vi "multichat.vi"() -> ()   [LabVIEW 2016]
uses:
  <vilib>/httpClient/POSTBuffer.vi
  <vilib>/httpClient/LabVIEWHTTPClient.lvlib
panel:
  in  "AgentIds":string[](array[string])
  out "Error Msg":string
  out "OK?":bool
  out "Trancscript":string
  in  "User Text":string
  out "error out":errorcluster
  in  "error in":errorcluster
  in  "Base URL":string="http://localhost:3000"
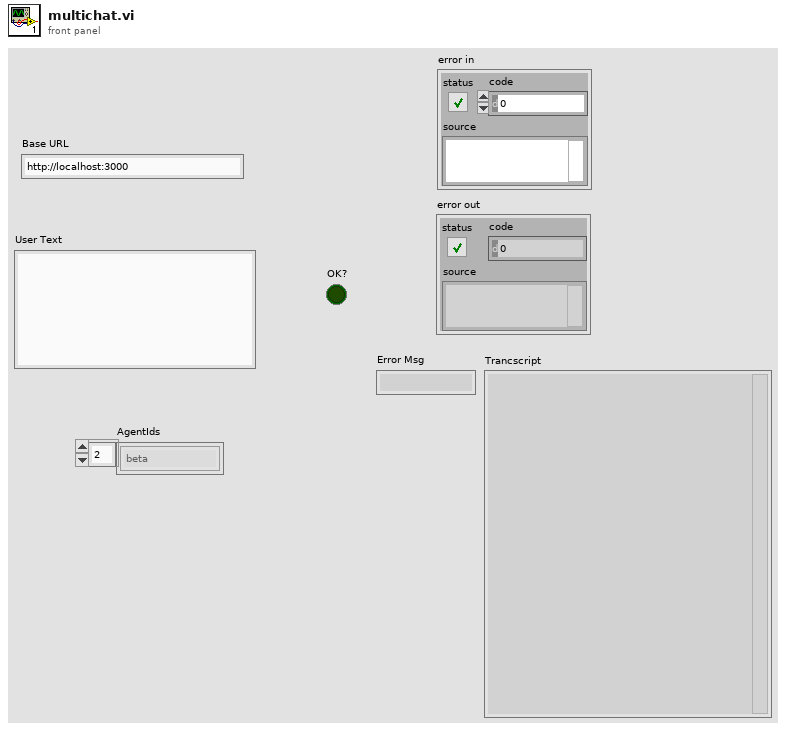
[diagram p1: front panel]
types:
  T1 = cluster{"ok":bool, "transcript":string, "error":string}
  T2 = typedef "LabVIEWHTTPClient.lvlib/ClientHandle.ctl" = refnum<k1>
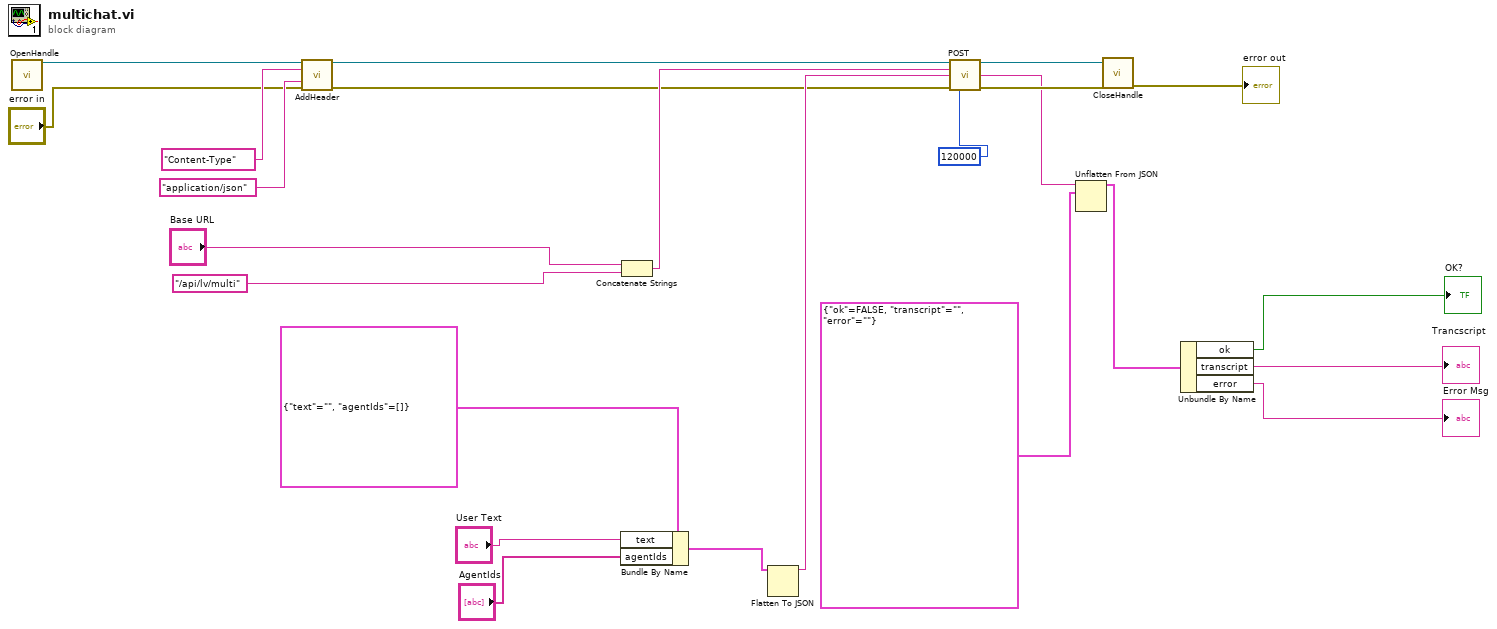
[diagram p0: block diagram]
diagram:
  n1 = call <vilib>:"OpenHandle.vi"() -> ("client handle out"=w22:T2)  [unwired: 14 in, 1 out]
  n2 = call <vilib>:"AddHeader.vi"("client handle"=w22, "header"="Content-Type", "value"="application/json", "error in (no error)"="error in") -> ("client handle out"=w19:T2, "error out"=w14:errorcluster)  [unwired: 10 in]
  n3 = Bundle By Name(cluster=cluster{"text":string, "agentIds":string[]} {"text"="", "agentIds"=[]}, "text"="User Text", "agentIds"="AgentIds") -> (w6:cluster{"text":string, "agentIds":string[]})
  n4 = Concatenate Strings("Base URL", "/api/lv/multi") -> (w18:string)
  n5 = Flatten To JSON(anything=w6) -> (JSON string=w17:string)  [unwired: 2 in, 1 out]
  n6 = call-poly <vilib>:"POST.vi"("client handle"=w19, "url"=w18, "buffer"=w17, "error in (no error)"=w14, "timeout (10000)"=120000) -> ("client handle out"=w16:T2, "body"=w12:string, "error out"=w13:errorcluster)  [unwired: 7 in, 1 out]
  n7 = Unflatten From JSON(JSON string=w12, type and defaults=T1 {"ok"=FALSE, "transcript"="", "error"=""}) -> (value=w4:T1)  [unwired: 5 in, 1 out]
  n8 = call <vilib>:"CloseHandle.vi"("client handle"=w16, "error in (no error)"=w13) -> ("error out"=→"error out":errorcluster)  [unwired: 13 in]
  n9 = Unbundle By Name(w4) -> ("ok"=→"OK?":bool, "transcript"=→"Trancscript":string, "error"=→"Error Msg":string)
